vi "Get Self Alias.vi"(11 "Sender in":refnum<class "Sender.lvclass">) -> (2 "Self Alias":string)   [LabVIEW 2021, in "jettl.lvlib" / "Sender.lvlib" / "Sender.lvclass"]
uses:
  Sender.lvclass
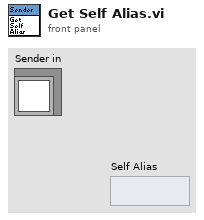
[diagram p1: front panel]
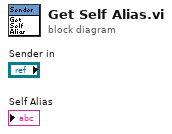
[diagram p0: block diagram]
diagram:
